vi "My_RIGOL_v1_3_different_vi.vi"(0 "VISA":refnum<visa-resource-name>, 1 "Amplitude Unit (0: Vpp)":i32(ring) items=["Vpp", "Vrms", "dBm"], 2 "Частота (1000 Hz)":dbl=1000.0 format="%#_12p", 3 "Сколько точек\n сдвигать":i32, 6 "Amplitude Диода (5 Vpp) 2":dbl=5.0, 8 "Количество точек":dbl, 10 "Amplitude Детектора (5 Vpp)":dbl=5.0, 12 "Amplitude Unit (0: Vpp) 2":i32(ring) items=["Vpp", "Vrms", "dBm"], 14 "Коэффициент амплитуды":dbl format="%#_12f", 15 "Точек между импульсами, тчк":dbl format="%#_12p", 16 "Ширина импульса, тчк":dbl=1000.0 format="%#_12p", 17 "Ширина импульса, с 2":dbl=1000.0 format="%#_12p", 18 "Время между импульсами, с 2":dbl format="%#_12p", 19 "Ширина отрицательного импульса, с":dbl=1000.0 format="%#_12p") -> (4 "Разница между \nсигналом диода и детектора, с":dbl format="%.12p", 5 "VISA resource name out":refnum<visa-resource-name>, 7 "Сигнал Детектора":cluster{"Y":dbl[], "Y":dbl[]}[](graph) caption="XY Graph 3", 9 "Сигнал Диода":cluster{"Y":dbl[], "Y":dbl[]}[](graph) caption="XY Graph 3", 11 "Выход на канал 1":string, 13 "Выход на канал 2":string)   [LabVIEW 2012]
panel:
  out "Начало интервала":string
  out "Оставшиеся точки":string
  out "Начало второго импульса":string
  out "Количество точек":string caption="String"
  out "Начало интервала":string
  out "Оставшиеся точки":string caption="String 3"
  out "Начало второго импульса":string
  out "Количество точек":string caption="String"
  # "Chanel 2"
  # "Chanel 1"
  # "ДИОД"
  # "ДЕТЕКТОР"
  # "ДЕТЕКТОР"
  # "ДИОД"
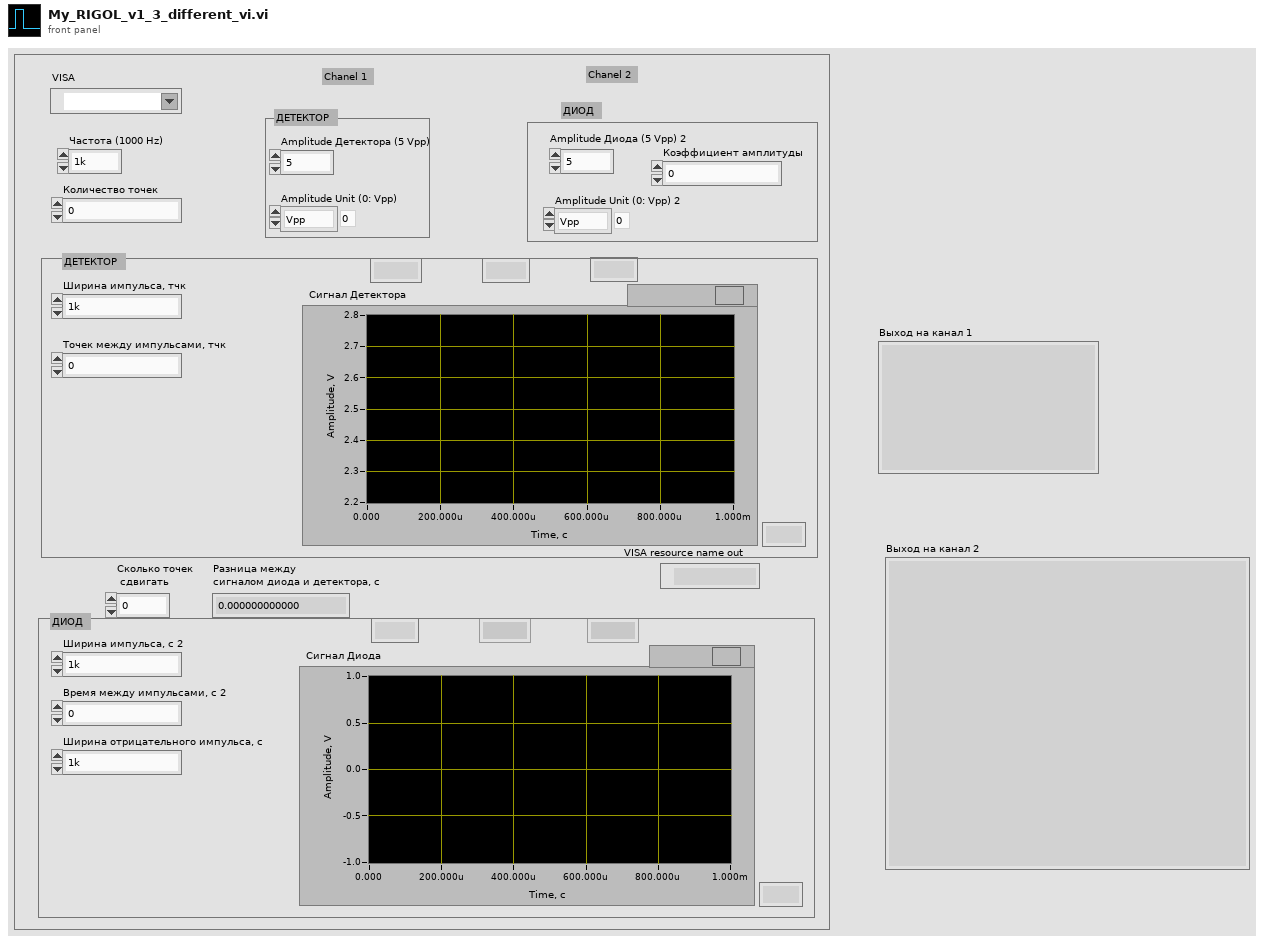
[diagram p1: front panel]
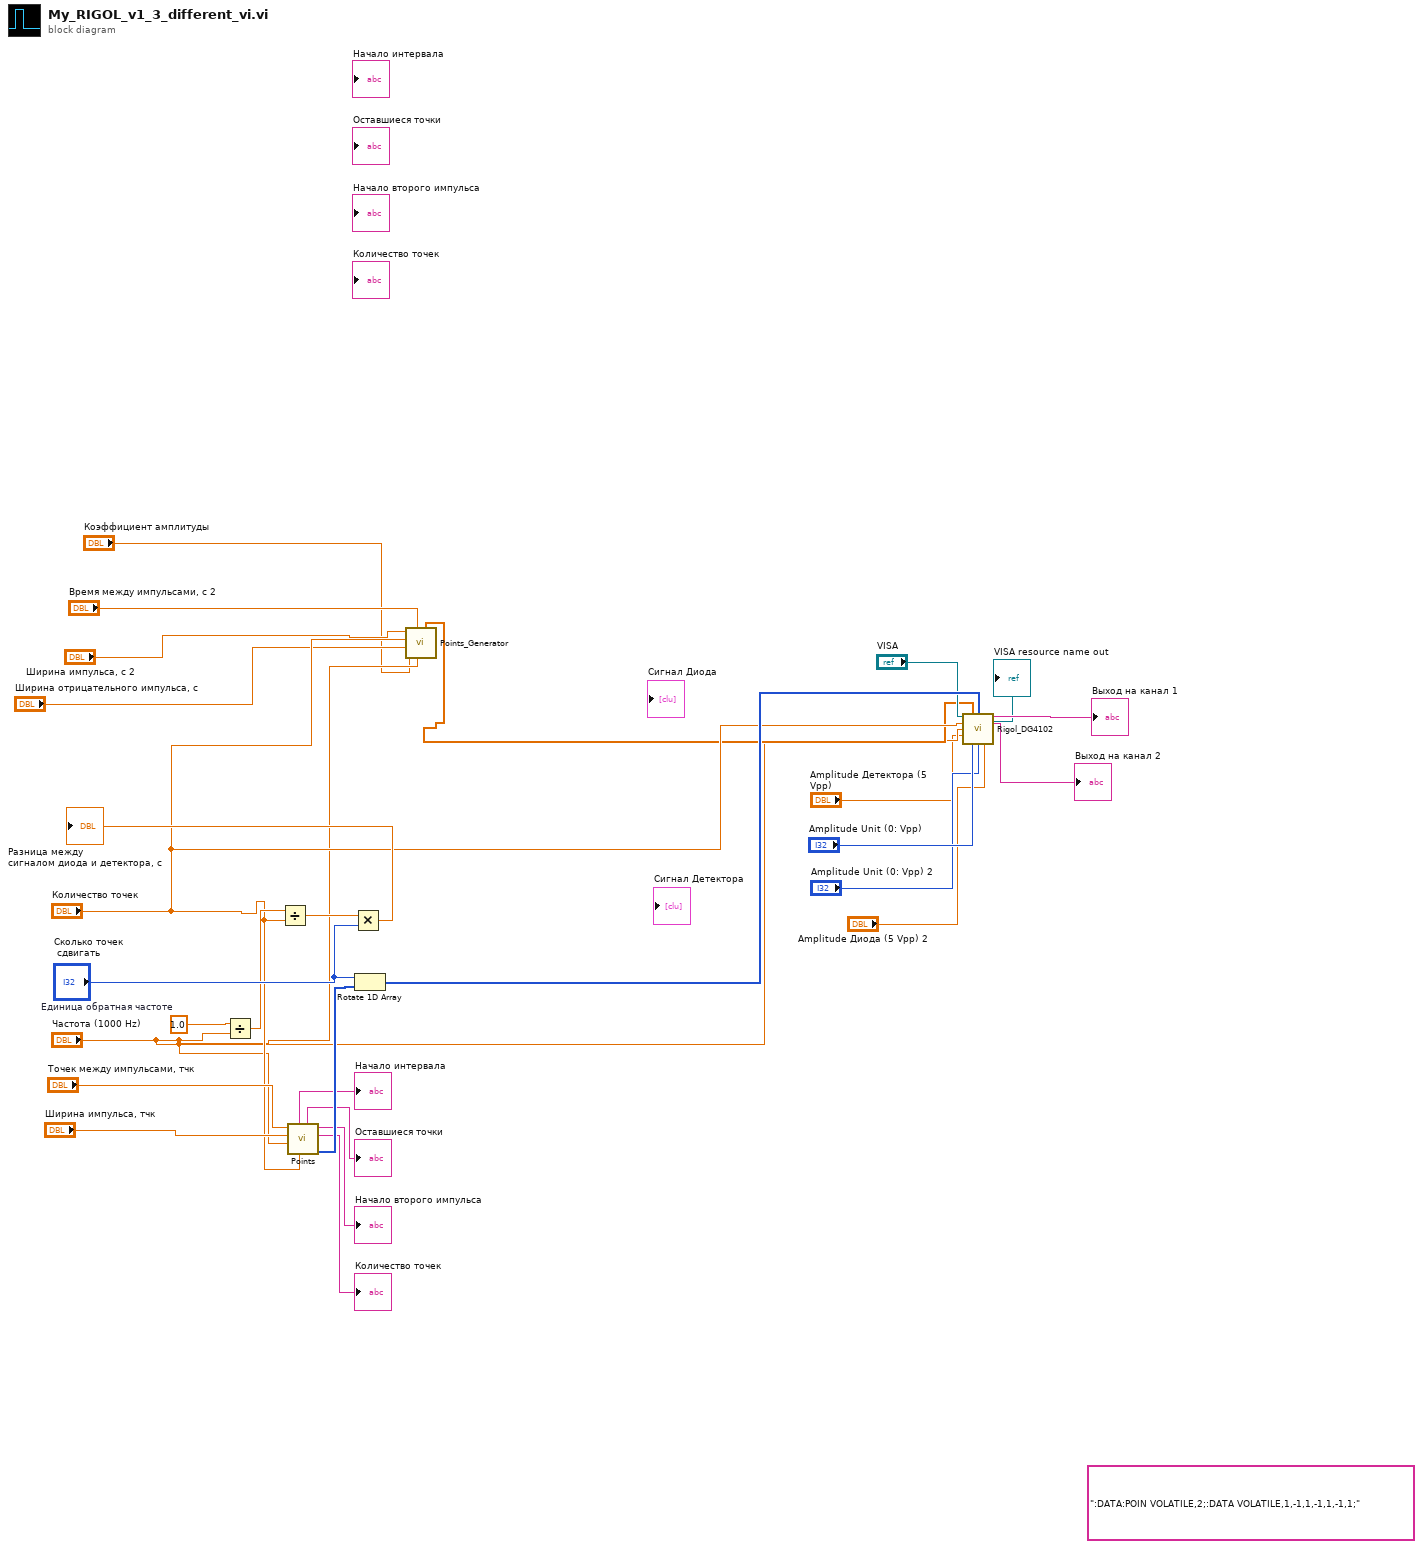
[diagram p0: block diagram]
diagram:
  w18 = 1.0  # Единица обратная частоте
  (unwired) ":DATA:POIN VOLATILE,2;:DATA VOLATILE,1,-1,1,-1,1,-1,1;"
  n1 = Divide(x=w18, y="Частота (1000 Hz)") -> (x/y=w19:dbl)
  n2 = Divide(x=w19, y="Количество точек") -> (x/y=w17:dbl)
  n3 = call "Points.vi"("Количество точек"="Количество точек", "Частота (1000 Hz)"="Частота (1000 Hz)", "Ширина импульса, тчк"="Ширина импульса, тчк", "Точек между импульсами, тчк"="Точек между импульсами, тчк") -> ("Детектор"=w24:i32[], "Количество точек"=→"Количество точек":string, "Начало второго импульса"=→"Начало второго импульса":string, "Оставшиеся точки"=→"Оставшиеся точки":string, "Начало интервала"=→"Начало интервала":string)  [unwired: 2 in, 1 out]
  n4 = Multiply(x=w17, y="Сколько точек\n сдвигать") -> (x*y=→"Разница между \nсигналом диода и детектора, с":dbl)
  n5 = Rotate 1D Array(1:w24, 2:"Сколько точек\n сдвигать") -> (0:w14:i32[])
  n6 = call "Points_Generator.vi"("Частота (1000 Hz)"="Частота (1000 Hz)", "Точек между импульсами, тчк in"="Время между импульсами, с 2", "Коэффициент амплитуды"="Коэффициент амплитуды", "Ширина отрицательного импульса, тчк in"="Ширина отрицательного импульса, с", "Количество точек in"="Количество точек", "Ширина импульса, тчк in"="Ширина импульса, с 2") -> ("Один импульс (диод)"=w7:dbl[])  [unwired: 5 out]
  n7 = call "Rigol_DG4102.vi"("VISA Refnum in"="VISA", "Массив диода"=w7, "Масиив детектора"=w14, "Количество точек"="Количество точек", "Частота (1000 Hz)"="Частота (1000 Hz)", "Amplitude (5 Vpp)"="Amplitude Детектора (5 Vpp)", "Amplitude Unit (0: Vpp)"="Amplitude Unit (0: Vpp)", "Amplitude Unit (0: Vpp) 2"="Amplitude Unit (0: Vpp) 2", "Amplitude (5 Vpp) 2"="Amplitude Диода (5 Vpp) 2") -> ("VISA resource name out"=→"VISA resource name out":refnum<visa-resource-name>, "Выход на канал 1"=→"Выход на канал 1":string, "Выход на канал 2"=→"Выход на канал 2":string)  [unwired: 4 in]
